vi "Construct_Bad_Track_Except_(11-111)_Point-3.vi"(6 "[IN] Indexes for Jumps":i32[](array[numeric]), 8 "error IN":errorcluster, 9 "[IN] Index of recon\nstructed tracks":i32, 10 "[IN] Clusters for Re\nconstructed Tracks":T1, 11 "[IN] Still connected\ntracks in group":T2) -> (0 "error OUT":errorcluster, 2 "[OUT] Clusters for Re\nconstructed Tracks":T1)   [LabVIEW 2013]
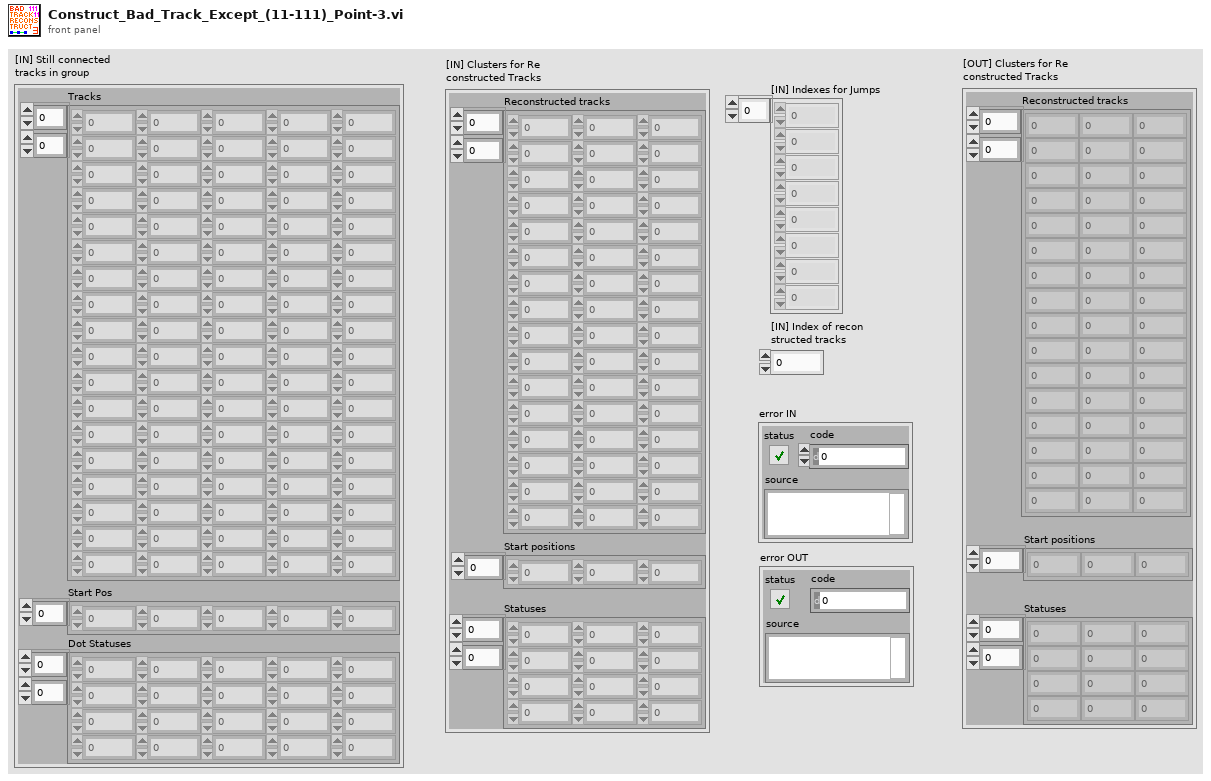
[diagram p1: front panel]
types:
  T1 = cluster{"Reconstructed tracks":dbl[][], "Start positions":i32[], "Statuses":i16[][]}
  T2 = cluster{"Tracks":dbl[][], "Start Pos":i32[], "Dot Statuses":i16[][]}
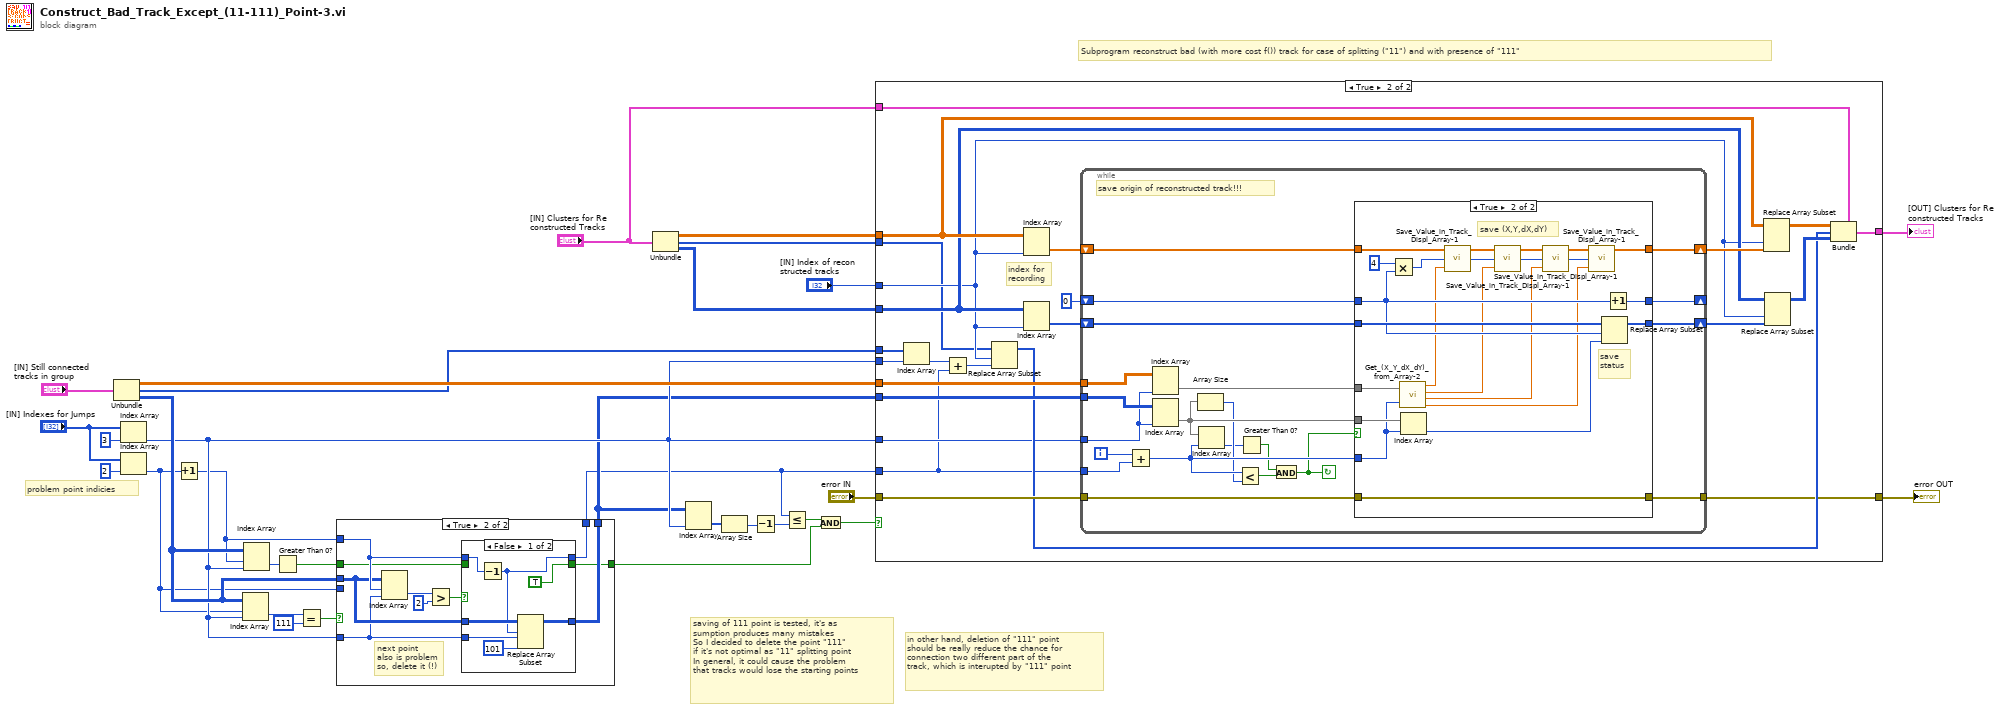
[diagram p0: block diagram]
diagram:
  # "in other hand, deletion of \"111\" point \nshould be really reduce the chance for\nconnection two different part of the \ntrack, which is interupted by \"111\" point"
  # "saving of 111 point is tested, it's as\nsumption produces many mistakes\nSo I decided to delete the point \"111\"\nif it's not optimal as \"11\" splitting point\nIn general, it could cause the problem\nthat tracks would lose the starting points"
  # "problem point indicies"
  # "Subprogram reconstruct bad (with more cost f()) track for case of splitting (\"11\") and with presence of \"111\""
  n1 = Unbundle("[IN] Still connected\ntracks in group") -> ("Tracks"=w27:dbl[][], "Start Pos"=w13:i32[], "Dot Statuses"=w9:i16[][])
  n2 = Index Array(array="[IN] Indexes for Jumps", index=3) -> (element=w8:i32)
  n3 = Index Array(array="[IN] Indexes for Jumps", index=2) -> (element=w7:i32)
  n4 = Increment(x=w7) -> (x+1=w2:i32)
  n5 = Index Array(array=w9, index (row)=w7, index (col)=w8) -> (element=w11:i16)
  n6 = Index Array(array=w9, index (row)=w2, index (col)=w8) -> (element=w22:i16)
  n7 = Greater Than 0?(x=w22) -> (x > 0?=w4:bool)
  n8 = Equal?(x=w11, y=i16 111) -> (x = y?=w1:bool)
  n9 = case shown="True" w1 {
    tunnel: w9 -> [w32 w39]
    tunnel: w8 -> [_ w35]
    tunnel: w7 -> [_ _]
    tunnel: [w32 w38] -> w6
    tunnel: [w34 w36] -> w5
    tunnel: w4 -> [w34 w37]
    tunnel: [w33 w40] -> w3
    tunnel: w2 -> [w33 w41]
    frame False {
    }
    frame True {
      # "next point\nalso is problem\nso, delete it (!)"
      n10 = Index Array(array=w39, index (row)=w41, index (col)=w35) -> (element=w44:i16)
      n11 = Greater?(x=w44, y=i16 2) -> (0:w42:bool)
      n12 = case shown="False" w42 {
        tunnel: w41 -> [w51 w54]
        tunnel: [w47 w54] -> w40
        tunnel: w39 -> [w49 w53]
        tunnel: [w48 w53] -> w38
        tunnel: w37 -> [_ w52]
        tunnel: [TRUE w52] -> w36
        tunnel: w35 -> [w46 _]
        frame False {
          n13 = Decrement(x=w51) -> (x-1=w47:i32)
          n14 = Replace Array Subset(array=w49, new element=i16 101 ("new element/subarray"), index (row)=w47, index (col)=w46) -> (w48:i16[][])
        }
        frame True {
        }
      }
    }
  }
  n15 = Unbundle("[IN] Clusters for Re\nconstructed Tracks") -> ("Reconstructed tracks"=w26:dbl[][], "Start positions"=w12:i32[], "Statuses"=w25:i16[][])
  n16 = Index Array(array=w6, index (col)=w8) -> (element=w21:i16[])  [unwired: 1 in]
  n17 = Array Size(array=w21) -> (size(s)=w20:i32)
  n18 = Decrement(x=w20) -> (x-1=w19:i32)
  n19 = Less Or Equal?(x=w3, y=w19) -> (x <= y?=w18:bool)
  n20 = And(x=w18, y=w5) -> (x .and. y?=w17:bool)
  n21 = case shown="True" w17 {
    tunnel: w27 -> [_ w77]
    tunnel: w26 -> [_ w70]
    tunnel: w25 -> [_ w69]
    tunnel: "[IN] Index of recon\nstructed tracks" -> [_ w64]
    tunnel: "error IN" -> [w55 w76]
    tunnel: w6 -> [_ w75]
    tunnel: "[IN] Clusters for Re\nconstructed Tracks" -> [w56 w71]
    tunnel: w13 -> [_ w65]
    tunnel: w8 -> [_ w67]
    tunnel: w3 -> [_ w59]
    tunnel: [w56 w61] -> w14
    tunnel: w8 -> [_ w60]
    tunnel: [w55 w58] -> w15
    tunnel: w12 -> [_ w57]
    frame False {
    }
    frame True {
      # "index for\nrecording"
      n22 = Index Array(array=w65, index=w67) -> (element=w66:i32)
      n23 = Add(x=w66, y=w59) -> (x+y=w63:i32)
      n24 = Replace Array Subset(array=w57, new element=w63, index=w64) -> (w62:i32[])
      n25 = Index Array(array=w70, index (col)=w64) -> (element=w80:dbl[])  [unwired: 1 in]
      n26 = Index Array(array=w69, index (col)=w64) -> (element=w79:i16[])  [unwired: 1 in]
      n27 = while {
        tunnel: w59 -> [w88]
        tunnel: w77 -> [w101]
        tunnel: w75 -> [w100]
        tunnel: w60 -> [w99]
        shift-right: [w94] -> w72
        shift-left: w80 -> [w98]
        shift-right: [w92] -> w68
        shift-left: w79 -> [w96]
        shift-right: [w93] -> _
        shift-left: 0 -> [w95]
        tunnel: w76 -> [w91]
        tunnel: [w90] -> w58
        i -> [w89]
        stop <- w81 continue-if-true
        # "save origin of reconstructed track!!!"
        n28 = Add(x=w89, y=w88) -> (x+y=w87:i32)
        n29 = Index Array(array=w101, index (col)=w99) -> (element=w97:dbl[])  [unwired: 1 in]
        n30 = Index Array(array=w100, index (col)=w99) -> (element=w86:i16[])  [unwired: 1 in]
        n31 = Array Size(array=w86) -> (size(s)=w85:i32)
        n32 = Index Array(array=w86, index=w87) -> (element=w83:i16)
        n33 = Less?(x=w87, y=w85) -> (x < y?=w82:bool)
        n34 = Greater Than 0?(x=w83) -> (x > 0?=w84:bool)
        n35 = And(x=w84, y=w82) -> (x .and. y?=w81:bool)
        n36 = case shown="True" w81 {
          tunnel: w98 -> [w105 w118]
          tunnel: w97 -> [_ w128]
          tunnel: w86 -> [_ w127]
          tunnel: w87 -> [_ w123]
          tunnel: w96 -> [w103 w125]
          tunnel: [w103 w122] -> w92
          tunnel: [w105 w106] -> w94
          tunnel: w95 -> [w104 w121]
          tunnel: [w104 w120] -> w93
          tunnel: w91 -> [w102 w119]
          tunnel: [w102 w119] -> w90
          frame False {
          }
          frame True {
            # "save (X,Y,dX,dY)"
            # "save\nstatus"
            n37 = Multiply(x=4, y=w121) -> (x*y=w117:i32)
            n38 = call "Get_(X_Y_dX_dY)_from_Array-2.vi"("(X,Y,dX,dY)"=w128, "Index of Displacement"=w123) -> ("X"=w116:dbl, "Y"=w113:dbl, "dX"=w110:dbl, "dY"=w107:dbl)
            n39 = Index Array(array=w127, index=w123) -> (element=w124:i16)
            n40 = call "Save_Value_in_Track_Displ_Array-1.vi"("[IN] Value"=w116, "[IN] Index"=w117, "[IN] Empty tracks\nfor points saving"=w118) -> ("[OUT] Index ++"=w114:i32, "[OUT Track with saved value"=w115:dbl[])  [unwired: 1 in]
            n41 = call "Save_Value_in_Track_Displ_Array-1.vi"("[IN] Value"=w113, "[IN] Index"=w114, "[IN] Empty tracks\nfor points saving"=w115) -> ("[OUT] Index ++"=w111:i32, "[OUT Track with saved value"=w112:dbl[])  [unwired: 1 in]
            n42 = call "Save_Value_in_Track_Displ_Array-1.vi"("[IN] Value"=w110, "[IN] Index"=w111, "[IN] Empty tracks\nfor points saving"=w112) -> ("[OUT] Index ++"=w108:i32, "[OUT Track with saved value"=w109:dbl[])  [unwired: 1 in]
            n43 = call "Save_Value_in_Track_Displ_Array-1.vi"("[IN] Value"=w107, "[IN] Index"=w108, "[IN] Empty tracks\nfor points saving"=w109) -> ("[OUT Track with saved value"=w106:dbl[])  [unwired: 1 in, 1 out]
            n44 = Replace Array Subset(array=w125, new element=w124, index=w121) -> (w122:i16[])
            n45 = Increment(x=w121) -> (x+1=w120:i32)
          }
        }
      }
      n46 = Replace Array Subset(array=w70, new element=w72, index (col)=w64) -> (w73:dbl[][])  [unwired: 1 in]
      n47 = Replace Array Subset(array=w69, new element=w68, index (col)=w64) -> (w74:i16[][])  [unwired: 1 in]
      n48 = Bundle(cluster=w71, "Reconstructed tracks"=w73, "Start positions"=w62, "Statuses"=w74) -> (w61:T1)
    }
  }
  "[OUT] Clusters for Re\nconstructed Tracks" <- w14
  "error OUT" <- w15
